vi "PS Set current.vi"(6 "Ramp":bool, 7 "error In":errorcluster, 9 "SetPoint":dbl format="%.2f", 10 "VISA Resource Name":refnum<visa-resource-name>) -> (0 "error out":errorcluster, 1 "Update?":bool, 3 "dup VISA Resource Name":refnum<visa-resource-name>, 4 "SetPoint Out":dbl format="%.2f")   [LabVIEW 2020]
uses:
  Serial Support VISA.llb/Serial Actions.ctl
  PS Comm Globals.vi
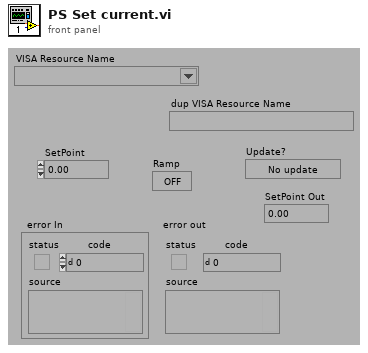
[diagram p1: front panel]
types:
  T1 = typedef "Serial Actions.ctl" = enum16{"Init", "Break", "Clear Buffer", "Write", "Read", "N Bytes", "Lock", "Unlock", "Close"}
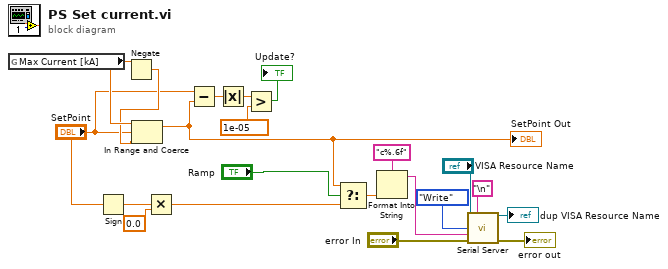
[diagram p0: block diagram]
diagram:
  n1 = global read "PS Comm Globals.vi" "Max Current [kA]"() -> (w10:dbl)
  n2 = Sign(1:"SetPoint") -> (0:w12:dbl)
  n3 = Negate(x=w10) -> (-x=w9:dbl)
  n4 = In Range and Coerce(upper limit=w10, x="SetPoint", lower limit=w9) -> (coerced(x)=w2:dbl)  [unwired: 1 out]
  "SetPoint Out" <- w2
  n5 = Multiply(x=w12, y=0.0 ("x")) -> (x*y=w11:dbl)
  n6 = Subtract(x="SetPoint", y=w2) -> (x-y=w17:dbl)
  n7 = Absolute Value(x=w17) -> (abs(x)=w15:dbl)
  n8 = Greater?(x=w15, y=1e-05) -> (0:→"Update?":bool)
  n9 = Select(t=w2, s="Ramp", f=w11) -> (s? t:f=w3:dbl)
  n10 = Format Into String(format string="c%.6f", w3) -> (resulting string=w4:string)  [unwired: 2 in, 1 out]
  n11 = call "Serial Server.vi"("VISA Resource Name"="VISA Resource Name", "EOT Chars (cr/lf)"="\n", "Action"=Serial_Actions."Write", "String To Send"=w4, "error in (no error)"="error In") -> ("dup VISA Resource Name"=→"dup VISA Resource Name":refnum<visa-resource-name>, "error out"=→"error out":errorcluster)  [unwired: 6 in, 3 out]
